vi "Fetch Multiple Measurements (Current Data).vi"(0 "VISA resource name":refnum<visa-resource-name>, 11 "error in (no error)":errorcluster) -> (4 "VISA resource name out":refnum<visa-resource-name>, 6 "Instantaneous Current":dbl[](array[numeric]), 8 "Current Harmonic Amplitudes":dbl[](array[numeric]), 10 "Current Harmonic Phase Angles":dbl[](array[numeric]), 15 "error out":errorcluster)   [LabVIEW 2020, in "Agilent 681x Series.lvlib"]
doc: "Fetches and returns the last 4096 instantaneous current measurements, the first 50 harmonic amplitudes and phase values.\n\n<B>Note:</B>\n\nUse this VI only with other low-level VIs. The high-level VIs automatically incorporate this functionality. This VI does not check the instrument status. If you want to check the instrument status, call the Error Query VI at the conclusion of the sequence."
uses:
  <instrlib>/Agilent 681x Series/Agilent 681x Series.lvlib
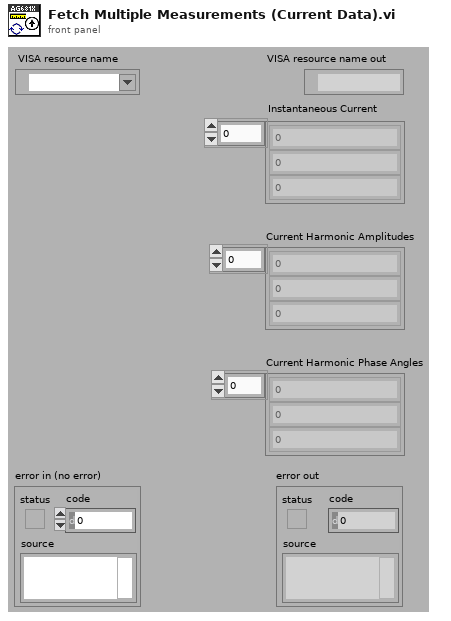
[diagram p1: front panel]
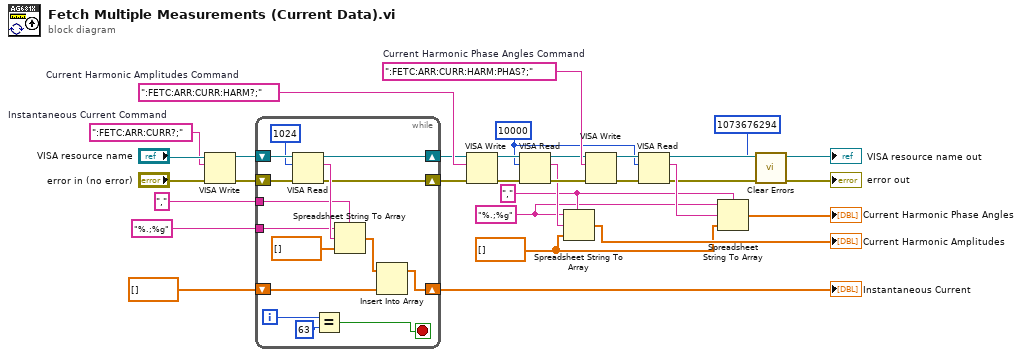
[diagram p0: block diagram]
diagram:
  w2 = dbl[] []
  w5 = "," ("format string")
  w4 = "%.;%g" ("format string")
  w16 = u32 10000 ("byte count")
  w22 = ":FETC:ARR:CURR:HARM:PHAS?;"  # Current Harmonic Phase Angles Command
  w23 = ":FETC:ARR:CURR:HARM?;"  # Current Harmonic Amplitudes Command
  w27 = ":FETC:ARR:CURR?;"  # Instantaneous Current Command
  n1 = VISA Write(VISA resource name="VISA resource name", write buffer=w27, error in (no error)="error in (no error)") -> (VISA resource name out=w28:refnum<visa-resource-name>, error out=w29:errorcluster)  [unwired: 1 out]
  n2 = while {
    shift-right: [w42] -> w15
    shift-left: w29 -> [w46]
    shift-right: [w41] -> w14
    shift-left: w28 -> [w45]
    shift-right: [w39] -> w13
    shift-left: dbl[] [] -> [w37]
    tunnel: "," ("format string") -> [w33]
    tunnel: "%.;%g" ("format string") -> [w32]
    i -> [w36]
    stop <- w34 stop-if-true
    n3 = VISA Read(VISA resource name=w45, byte count=u32 1024, error in (no error)=w46) -> (VISA resource name out=w41:refnum<visa-resource-name>, read buffer=w43:string, error out=w42:errorcluster)  [unwired: 1 out]
    n4 = Equal?(x=w36, y=63) -> (x = y?=w34:bool)
    n5 = Spreadsheet String To Array(delimiter (Tab)=w33, format string=w32, spreadsheet string=w43, array type (2D Dbl)=dbl[] []) -> (array=w38:dbl[])
    n6 = Insert Into Array(array=w38, new element=w37) -> (w39:dbl[])  [unwired: 1 in]
  }
  "Instantaneous Current" <- w13
  n7 = VISA Write(VISA resource name=w14, write buffer=w23, error in (no error)=w15) -> (VISA resource name out=w21:refnum<visa-resource-name>, error out=w25:errorcluster)  [unwired: 1 out]
  n8 = VISA Read(VISA resource name=w21, byte count=w16, error in (no error)=w25) -> (VISA resource name out=w20:refnum<visa-resource-name>, read buffer=w9:string, error out=w26:errorcluster)  [unwired: 1 out]
  n9 = Spreadsheet String To Array(delimiter (Tab)=w5, format string=w4, spreadsheet string=w9, array type (2D Dbl)=w2) -> (array=→"Current Harmonic Amplitudes":dbl[])
  n10 = VISA Write(VISA resource name=w20, write buffer=w22, error in (no error)=w26) -> (VISA resource name out=w19:refnum<visa-resource-name>, error out=w24:errorcluster)  [unwired: 1 out]
  n11 = VISA Read(VISA resource name=w19, byte count=w16, error in (no error)=w24) -> (VISA resource name out=→"VISA resource name out":refnum<visa-resource-name>, read buffer=w17:string, error out=w8:errorcluster)  [unwired: 1 out]
  n12 = Spreadsheet String To Array(delimiter (Tab)=w5, format string=w4, spreadsheet string=w17, array type (2D Dbl)=w2) -> (array=→"Current Harmonic Phase Angles":dbl[])
  n13 = call <vilib>:"Clear Errors.vi"("error in (no error)"=w8, "specific error code to clear (0: all)"=1073676294) -> ("error out"=→"error out":errorcluster)  [unwired: 4 in, 1 out]
